vi "SetTemp.vi"(1 "level 0..7":u32=1) -> ()   [LabVIEW 2014]
uses:
  ESLSCDLL.dll
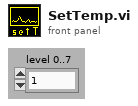
[diagram p1: front panel]
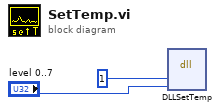
[diagram p0: block diagram]
diagram:
  n1 = dll-call lib="C:/Users/Gerhard/Documents/New64/lv/1cam/board.vis/ESLSCDLL.dll" fn="DLLSetTemp"("drv"=u32 1, "level"="level 0..7") -> ()  [unwired: 6 in, 2 out]
